vi "Write Coded Binary Data.vi"(7 "AC Data":refnum<class "Data.lvclass">, 8 "error in":errorcluster, 9 "cell":i32=-1, 10 "binRefIn":refnum<file>, 11 "PAS Cell Data in":refnum<class "PAS Cell Data.lvclass">) -> (0 "error out":errorcluster, 3 "PAS Cell Data out":refnum<class "PAS Cell Data.lvclass">)   [LabVIEW 2014, in "PAS Cell Data.lvclass"]
uses:
  PAS Cell Data.lvclass
  Data/Data.lvclass
  Main/Controls/Cell Data.ctl
  <vilib>/Analysis/Matrix/NI_Matrix.lvlib
  <vilib>/Analysis/Matrix/Numeric/Conversions/Matrix To Array - RM.vi
  Devices/Alicat/Data/MC/AlicatMCData.lvclass
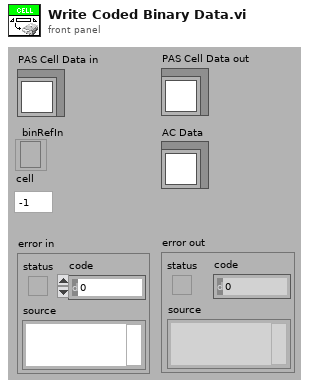
[diagram p1: front panel]
types:
  T1 = typedef "Cell Data.ctl" = u8
  T2 = enum16{"big-endian, network order", "native, host order", "little-endian"}
  T3 = typedef "NI_Matrix.lvlib/RealMatrix.ctl" = dbl[][]
  T4 = cluster{"P":sgl, "T":sgl, "Q":sgl, "Q0":sgl, "Qsp":sgl}
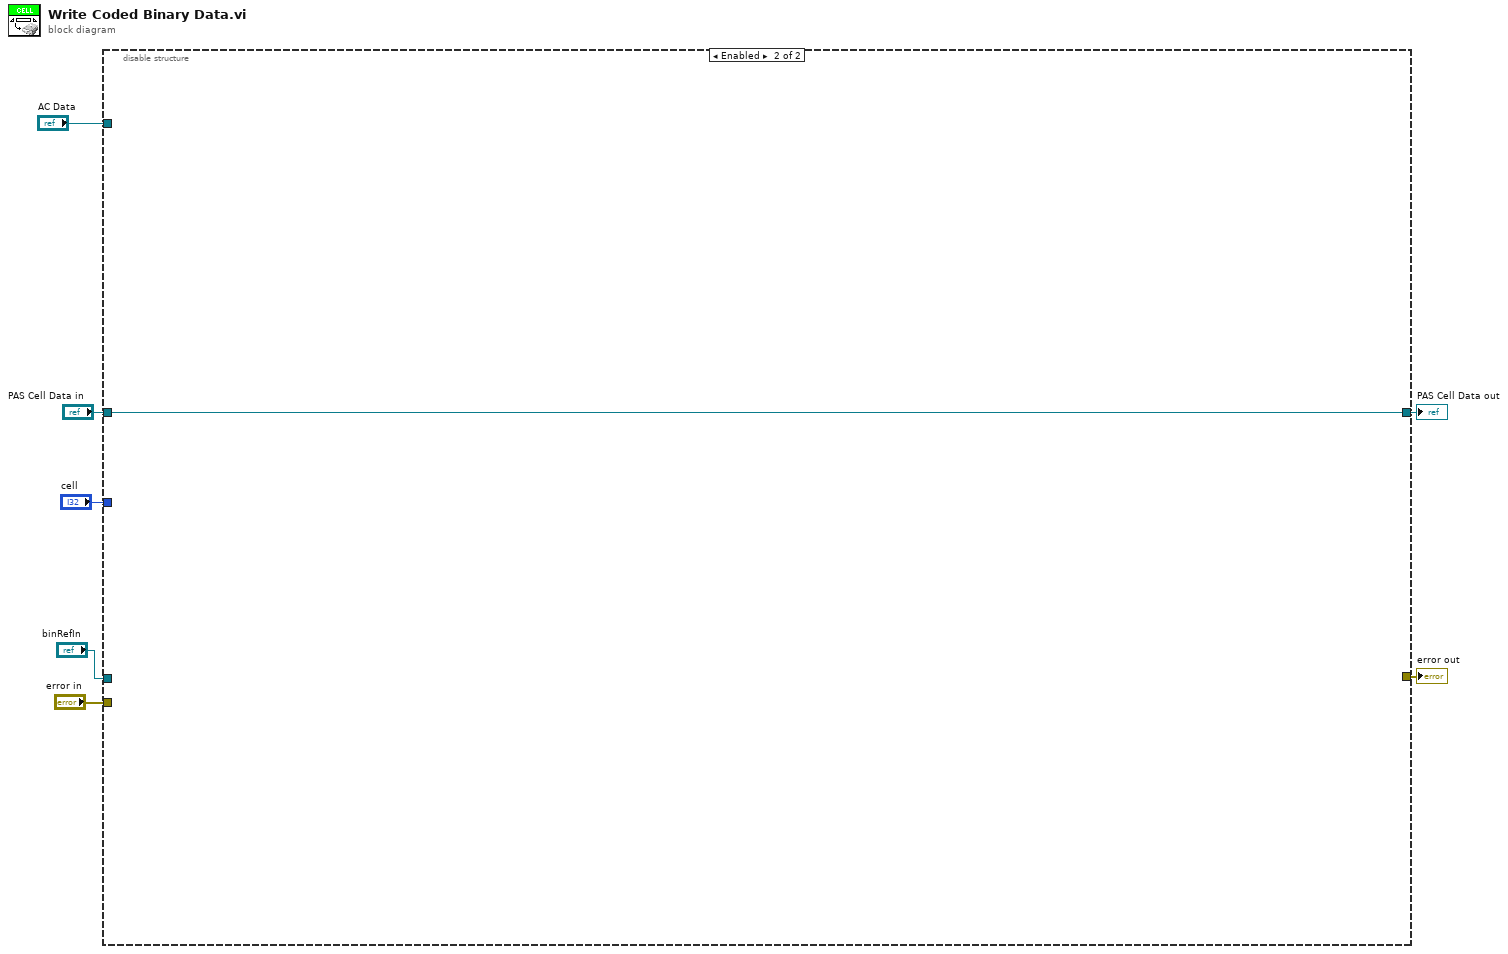
[diagram p0: block diagram]
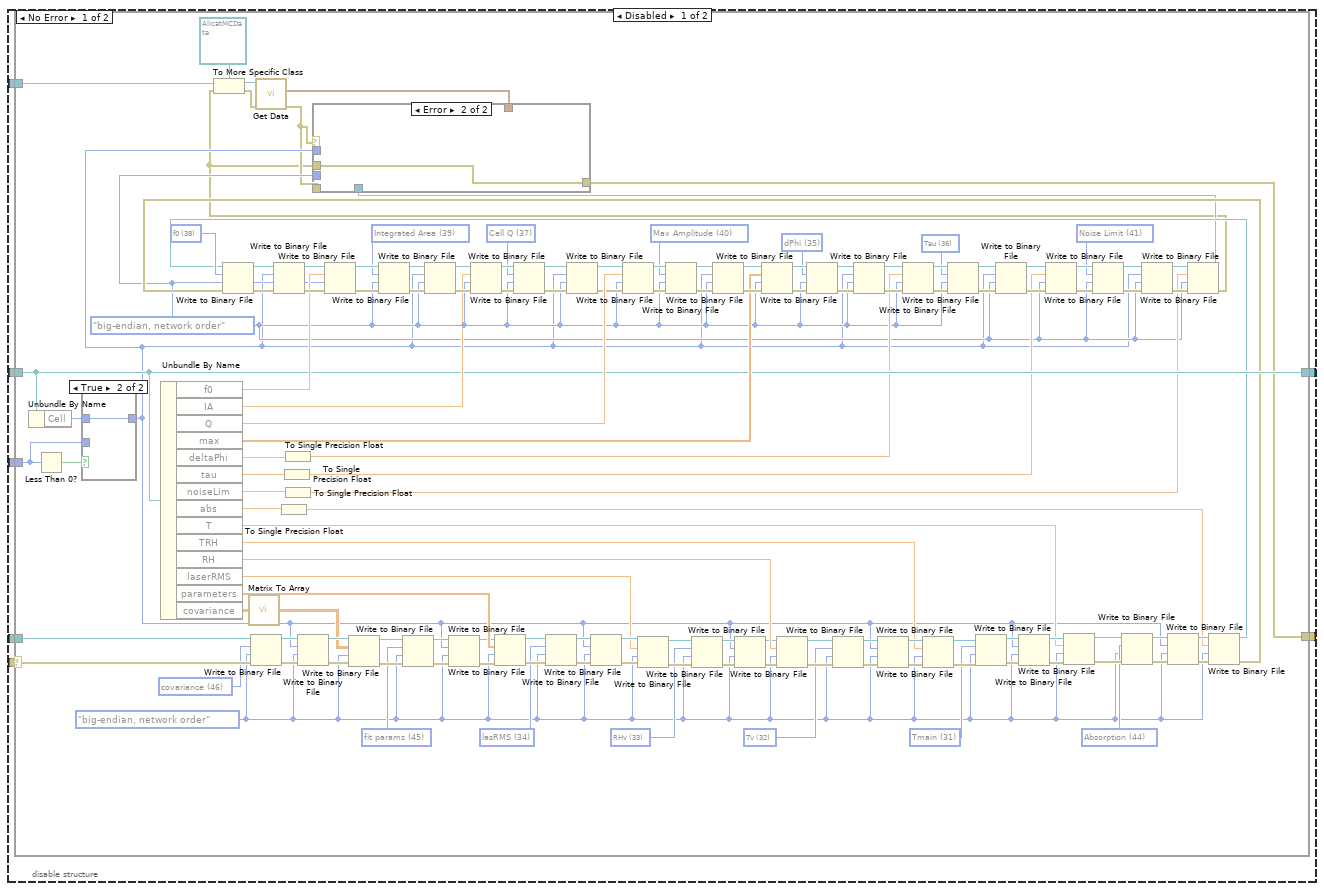
[diagram p2: hidden frame]
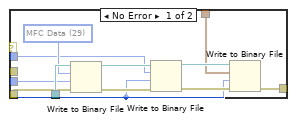
[diagram p3: hidden frame]
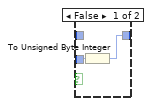
[diagram p4: hidden frame]
diagram:
  n1 = disable-structure shown="Enabled" {
    disable-tunnel: "error in" -> [w14 _]
    disable-tunnel: [w13 _] -> w6
    disable-tunnel: "PAS Cell Data in" -> [w12 w165]
    disable-tunnel: [w11 w165] -> w4
    disable-tunnel: "binRefIn" -> [w10 _]
    disable-tunnel: "cell" -> [w9 _]
    disable-tunnel: "AC Data" -> [w8 _]
    frame Disabled {
      n2 = case shown="No Error" w14 {
        selector: w14 -> [w147 w164]
        tunnel: [w19 w164] -> w13
        tunnel: [w39 w163] -> w11
        tunnel: w12 -> [w39 w163]
        tunnel: w10 -> [w55 _]
        tunnel: w9 -> [w27 _]
        tunnel: w8 -> [w24 _]
        frame No Error {
          w44 = T1 41 items=["TEC SP"=23, "TEC Enable"=24, "Qsp"=25, "Tac"=26, "Pac"=27, "Q0ac"=28, "Qac"=29, "Cell TEC T (T1)"=30, "Tmain"=31, "Tv"=32, "RHv"=33, "lasRMS"=34, "dPhi"=35, "Tau"=36, "Cell Q"=37, "f0"=38, "Integrated Area"=39, "Max Amplitude"=40, "Noise Limit"=41, "Lower Noise Bound"=42, "Upper Noise Bound"=43, "Absorption"=44, "fit params"=45, "covariance"=46] ("cellNumData")
          w45 = T1 36 items=["TEC SP"=23, "TEC Enable"=24, "Qsp"=25, "Tac"=26, "Pac"=27, "Q0ac"=28, "Qac"=29, "Cell TEC T (T1)"=30, "Tmain"=31, "Tv"=32, "RHv"=33, "lasRMS"=34, "dPhi"=35, "Tau"=36, "Cell Q"=37, "f0"=38, "Integrated Area"=39, "Max Amplitude"=40, "Noise Limit"=41, "Lower Noise Bound"=42, "Upper Noise Bound"=43, "Absorption"=44, "fit params"=45, "covariance"=46] ("cellNumData")
          w46 = T1 35 items=["TEC SP"=23, "TEC Enable"=24, "Qsp"=25, "Tac"=26, "Pac"=27, "Q0ac"=28, "Qac"=29, "Cell TEC T (T1)"=30, "Tmain"=31, "Tv"=32, "RHv"=33, "lasRMS"=34, "dPhi"=35, "Tau"=36, "Cell Q"=37, "f0"=38, "Integrated Area"=39, "Max Amplitude"=40, "Noise Limit"=41, "Lower Noise Bound"=42, "Upper Noise Bound"=43, "Absorption"=44, "fit params"=45, "covariance"=46] ("cellNumData")
          w48 = T1 40 items=["TEC SP"=23, "TEC Enable"=24, "Qsp"=25, "Tac"=26, "Pac"=27, "Q0ac"=28, "Qac"=29, "Cell TEC T (T1)"=30, "Tmain"=31, "Tv"=32, "RHv"=33, "lasRMS"=34, "dPhi"=35, "Tau"=36, "Cell Q"=37, "f0"=38, "Integrated Area"=39, "Max Amplitude"=40, "Noise Limit"=41, "Lower Noise Bound"=42, "Upper Noise Bound"=43, "Absorption"=44, "fit params"=45, "covariance"=46] ("cellNumData")
          w50 = T1 37 items=["TEC SP"=23, "TEC Enable"=24, "Qsp"=25, "Tac"=26, "Pac"=27, "Q0ac"=28, "Qac"=29, "Cell TEC T (T1)"=30, "Tmain"=31, "Tv"=32, "RHv"=33, "lasRMS"=34, "dPhi"=35, "Tau"=36, "Cell Q"=37, "f0"=38, "Integrated Area"=39, "Max Amplitude"=40, "Noise Limit"=41, "Lower Noise Bound"=42, "Upper Noise Bound"=43, "Absorption"=44, "fit params"=45, "covariance"=46] ("cellNumData")
          w52 = T1 39 items=["TEC SP"=23, "TEC Enable"=24, "Qsp"=25, "Tac"=26, "Pac"=27, "Q0ac"=28, "Qac"=29, "Cell TEC T (T1)"=30, "Tmain"=31, "Tv"=32, "RHv"=33, "lasRMS"=34, "dPhi"=35, "Tau"=36, "Cell Q"=37, "f0"=38, "Integrated Area"=39, "Max Amplitude"=40, "Noise Limit"=41, "Lower Noise Bound"=42, "Upper Noise Bound"=43, "Absorption"=44, "fit params"=45, "covariance"=46] ("cellNumData")
          w54 = T1 38 items=["TEC SP"=23, "TEC Enable"=24, "Qsp"=25, "Tac"=26, "Pac"=27, "Q0ac"=28, "Qac"=29, "Cell TEC T (T1)"=30, "Tmain"=31, "Tv"=32, "RHv"=33, "lasRMS"=34, "dPhi"=35, "Tau"=36, "Cell Q"=37, "f0"=38, "Integrated Area"=39, "Max Amplitude"=40, "Noise Limit"=41, "Lower Noise Bound"=42, "Upper Noise Bound"=43, "Absorption"=44, "fit params"=45, "covariance"=46] ("cellNumData")
          w18 = T2."big-endian, network order" ("byte order (0:big-endian, network order)")
          w93 = T1 44 items=["TEC SP"=23, "TEC Enable"=24, "Qsp"=25, "Tac"=26, "Pac"=27, "Q0ac"=28, "Qac"=29, "Cell TEC T (T1)"=30, "Tmain"=31, "Tv"=32, "RHv"=33, "lasRMS"=34, "dPhi"=35, "Tau"=36, "Cell Q"=37, "f0"=38, "Integrated Area"=39, "Max Amplitude"=40, "Noise Limit"=41, "Lower Noise Bound"=42, "Upper Noise Bound"=43, "Absorption"=44, "fit params"=45, "covariance"=46] ("cellNumData")
          w101 = T1 31 items=["TEC SP"=23, "TEC Enable"=24, "Qsp"=25, "Tac"=26, "Pac"=27, "Q0ac"=28, "Qac"=29, "Cell TEC T (T1)"=30, "Tmain"=31, "Tv"=32, "RHv"=33, "lasRMS"=34, "dPhi"=35, "Tau"=36, "Cell Q"=37, "f0"=38, "Integrated Area"=39, "Max Amplitude"=40, "Noise Limit"=41, "Lower Noise Bound"=42, "Upper Noise Bound"=43, "Absorption"=44, "fit params"=45, "covariance"=46] ("cellNumData")
          w109 = T1 32 items=["TEC SP"=23, "TEC Enable"=24, "Qsp"=25, "Tac"=26, "Pac"=27, "Q0ac"=28, "Qac"=29, "Cell TEC T (T1)"=30, "Tmain"=31, "Tv"=32, "RHv"=33, "lasRMS"=34, "dPhi"=35, "Tau"=36, "Cell Q"=37, "f0"=38, "Integrated Area"=39, "Max Amplitude"=40, "Noise Limit"=41, "Lower Noise Bound"=42, "Upper Noise Bound"=43, "Absorption"=44, "fit params"=45, "covariance"=46] ("cellNumData")
          w116 = T1 33 items=["TEC SP"=23, "TEC Enable"=24, "Qsp"=25, "Tac"=26, "Pac"=27, "Q0ac"=28, "Qac"=29, "Cell TEC T (T1)"=30, "Tmain"=31, "Tv"=32, "RHv"=33, "lasRMS"=34, "dPhi"=35, "Tau"=36, "Cell Q"=37, "f0"=38, "Integrated Area"=39, "Max Amplitude"=40, "Noise Limit"=41, "Lower Noise Bound"=42, "Upper Noise Bound"=43, "Absorption"=44, "fit params"=45, "covariance"=46] ("cellNumData")
          w125 = T1 34 items=["TEC SP"=23, "TEC Enable"=24, "Qsp"=25, "Tac"=26, "Pac"=27, "Q0ac"=28, "Qac"=29, "Cell TEC T (T1)"=30, "Tmain"=31, "Tv"=32, "RHv"=33, "lasRMS"=34, "dPhi"=35, "Tau"=36, "Cell Q"=37, "f0"=38, "Integrated Area"=39, "Max Amplitude"=40, "Noise Limit"=41, "Lower Noise Bound"=42, "Upper Noise Bound"=43, "Absorption"=44, "fit params"=45, "covariance"=46] ("cellNumData")
          w92 = T2."big-endian, network order" ("byte order (0:big-endian, network order)")
          w135 = T1 45 items=["TEC SP"=23, "TEC Enable"=24, "Qsp"=25, "Tac"=26, "Pac"=27, "Q0ac"=28, "Qac"=29, "Cell TEC T (T1)"=30, "Tmain"=31, "Tv"=32, "RHv"=33, "lasRMS"=34, "dPhi"=35, "Tau"=36, "Cell Q"=37, "f0"=38, "Integrated Area"=39, "Max Amplitude"=40, "Noise Limit"=41, "Lower Noise Bound"=42, "Upper Noise Bound"=43, "Absorption"=44, "fit params"=45, "covariance"=46] ("cellNumData")
          w145 = T1 46 items=["TEC SP"=23, "TEC Enable"=24, "Qsp"=25, "Tac"=26, "Pac"=27, "Q0ac"=28, "Qac"=29, "Cell TEC T (T1)"=30, "Tmain"=31, "Tv"=32, "RHv"=33, "lasRMS"=34, "dPhi"=35, "Tau"=36, "Cell Q"=37, "f0"=38, "Integrated Area"=39, "Max Amplitude"=40, "Noise Limit"=41, "Lower Noise Bound"=42, "Upper Noise Bound"=43, "Absorption"=44, "fit params"=45, "covariance"=46] ("cellNumData")
          n3 = Unbundle By Name(w39) -> ("Cell"=w26:u8)
          n4 = Less Than 0?(x=w27) -> (x < 0?=w28:bool)
          n5 = case shown="True" w28 {
            tunnel: w27 -> [w161 _]
            tunnel: [w160 w162] -> w17
            tunnel: w26 -> [_ w162]
            frame False {
              n6 = To Unsigned Byte Integer(number=w161) -> (unsigned 8bit integer=w160:u8)
            }
            frame True {
            }
          }
          n7 = Unbundle By Name(w39) -> ("f0"=w53:sgl, "IA"=w51:sgl, "Q"=w49:sgl, "max"=w47:dbl[], "deltaPhi"=w30:dbl, "tau"=w32:dbl, "noiseLim"=w34:dbl, "abs"=w36:dbl, "T"=w100:sgl, "TRH"=w108:sgl, "RH"=w123:sgl, "laserRMS"=w124:sgl, "parameters"=w134:dbl[], "covariance"=w146:T3)
          n8 = call-poly <vilib>:"Matrix To Array.vi"("Real Matrix"=w146) -> ("Real 2D Array"=w136:dbl[][])
          n9 = Write to Binary File(file (use dialog)=w55, data=w145, error in=w147, 9:w92) -> (refnum out=w143:refnum<file>, error out=w144:errorcluster)  [unwired: 2 in, 1 out]
          n10 = To Single Precision Float(number=w36) -> (single precision float=w35:sgl)
          n11 = To Single Precision Float(number=w32) -> (single precision float=w31:sgl)
          n12 = To Single Precision Float(number=w30) -> (single precision float=w29:sgl)
          n13 = To Single Precision Float(number=w34) -> (single precision float=w33:sgl)
          n14 = Write to Binary File(file (use dialog)=w143, data=w17, error in=w144, 9:w92) -> (refnum out=w142:refnum<file>, error out=w141:errorcluster)  [unwired: 2 in, 1 out]
          n15 = Write to Binary File(file (use dialog)=w142, data=w136, error in=w141, 9:w92) -> (refnum out=w140:refnum<file>, error out=w139:errorcluster)  [unwired: 2 in, 1 out]
          n16 = Write to Binary File(file (use dialog)=w140, data=w135, error in=w139, 9:w92) -> (refnum out=w138:refnum<file>, error out=w137:errorcluster)  [unwired: 2 in, 1 out]
          n17 = Write to Binary File(file (use dialog)=w138, data=w17, error in=w137, 9:w92) -> (refnum out=w133:refnum<file>, error out=w132:errorcluster)  [unwired: 2 in, 1 out]
          n18 = Write to Binary File(file (use dialog)=w133, data=w134, error in=w132, 9:w92) -> (refnum out=w131:refnum<file>, error out=w130:errorcluster)  [unwired: 2 in, 1 out]
          n19 = Write to Binary File(file (use dialog)=w131, data=w125, error in=w130, 9:w92) -> (refnum out=w129:refnum<file>, error out=w128:errorcluster)  [unwired: 2 in, 1 out]
          n20 = Write to Binary File(file (use dialog)=w129, data=w17, error in=w128, 9:w92) -> (refnum out=w127:refnum<file>, error out=w126:errorcluster)  [unwired: 2 in, 1 out]
          n21 = Write to Binary File(file (use dialog)=w127, data=w124, error in=w126, 9:w92) -> (refnum out=w122:refnum<file>, error out=w121:errorcluster)  [unwired: 2 in, 1 out]
          n22 = Write to Binary File(file (use dialog)=w122, data=w116, error in=w121, 9:w92) -> (refnum out=w120:refnum<file>, error out=w119:errorcluster)  [unwired: 2 in, 1 out]
          n23 = Write to Binary File(file (use dialog)=w120, data=w17, error in=w119, 9:w92) -> (refnum out=w118:refnum<file>, error out=w117:errorcluster)  [unwired: 2 in, 1 out]
          n24 = Write to Binary File(file (use dialog)=w118, data=w123, error in=w117, 9:w92) -> (refnum out=w114:refnum<file>, error out=w115:errorcluster)  [unwired: 2 in, 1 out]
          n25 = Write to Binary File(file (use dialog)=w114, data=w109, error in=w115, 9:w92) -> (refnum out=w112:refnum<file>, error out=w113:errorcluster)  [unwired: 2 in, 1 out]
          n26 = Write to Binary File(file (use dialog)=w112, data=w17, error in=w113, 9:w92) -> (refnum out=w110:refnum<file>, error out=w111:errorcluster)  [unwired: 2 in, 1 out]
          n27 = Write to Binary File(file (use dialog)=w110, data=w108, error in=w111, 9:w92) -> (refnum out=w106:refnum<file>, error out=w107:errorcluster)  [unwired: 2 in, 1 out]
          n28 = Write to Binary File(file (use dialog)=w106, data=w101, error in=w107, 9:w92) -> (refnum out=w105:refnum<file>, error out=w104:errorcluster)  [unwired: 2 in, 1 out]
          n29 = Write to Binary File(file (use dialog)=w105, data=w17, error in=w104, 9:w92) -> (refnum out=w103:refnum<file>, error out=w102:errorcluster)  [unwired: 2 in, 1 out]
          n30 = Write to Binary File(file (use dialog)=w103, data=w100, error in=w102, 9:w92) -> (refnum out=w99:refnum<file>, error out=w98:errorcluster)  [unwired: 2 in, 1 out]
          n31 = Write to Binary File(file (use dialog)=w99, data=w93, error in=w98, 9:w92) -> (refnum out=w97:refnum<file>, error out=w96:errorcluster)  [unwired: 2 in, 1 out]
          n32 = Write to Binary File(file (use dialog)=w97, data=w17, error in=w96, 9:w92) -> (refnum out=w95:refnum<file>, error out=w94:errorcluster)  [unwired: 2 in, 1 out]
          n33 = Write to Binary File(file (use dialog)=w95, data=w35, error in=w94, 9:w92) -> (refnum out=w38:refnum<file>, error out=w37:errorcluster)  [unwired: 2 in, 1 out]
          n34 = Write to Binary File(file (use dialog)=w38, data=w54, error in=w37, 9:w18) -> (refnum out=w57:refnum<file>, error out=w56:errorcluster)  [unwired: 2 in, 1 out]
          n35 = Write to Binary File(file (use dialog)=w57, data=w17, error in=w56, 9:w18) -> (refnum out=w58:refnum<file>, error out=w59:errorcluster)  [unwired: 2 in, 1 out]
          n36 = Write to Binary File(file (use dialog)=w58, data=w53, error in=w59, 9:w18) -> (refnum out=w60:refnum<file>, error out=w61:errorcluster)  [unwired: 2 in, 1 out]
          n37 = Write to Binary File(file (use dialog)=w60, data=w52, error in=w61, 9:w18) -> (refnum out=w62:refnum<file>, error out=w63:errorcluster)  [unwired: 2 in, 1 out]
          n38 = Write to Binary File(file (use dialog)=w62, data=w17, error in=w63, 9:w18) -> (refnum out=w64:refnum<file>, error out=w65:errorcluster)  [unwired: 2 in, 1 out]
          n39 = Write to Binary File(file (use dialog)=w64, data=w51, error in=w65, 9:w18) -> (refnum out=w66:refnum<file>, error out=w67:errorcluster)  [unwired: 2 in, 1 out]
          n40 = Write to Binary File(file (use dialog)=w66, data=w50, error in=w67, 9:w18) -> (refnum out=w42:refnum<file>, error out=w43:errorcluster)  [unwired: 2 in, 1 out]
          n41 = Write to Binary File(file (use dialog)=w42, data=w17, error in=w43, 9:w18) -> (refnum out=w41:refnum<file>, error out=w40:errorcluster)  [unwired: 2 in, 1 out]
          n42 = Write to Binary File(file (use dialog)=w41, data=w49, error in=w40, 9:w18) -> (refnum out=w68:refnum<file>, error out=w69:errorcluster)  [unwired: 2 in, 1 out]
          n43 = Write to Binary File(file (use dialog)=w68, data=w48, error in=w69, 9:w18) -> (refnum out=w70:refnum<file>, error out=w71:errorcluster)  [unwired: 2 in, 1 out]
          n44 = Write to Binary File(file (use dialog)=w70, data=w17, error in=w71, 9:w18) -> (refnum out=w72:refnum<file>, error out=w73:errorcluster)  [unwired: 2 in, 1 out]
          n45 = Write to Binary File(file (use dialog)=w72, data=w47, error in=w73, 9:w18) -> (refnum out=w74:refnum<file>, error out=w75:errorcluster)  [unwired: 2 in, 1 out]
          n46 = Write to Binary File(file (use dialog)=w74, data=w46, error in=w75, 9:w18) -> (refnum out=w77:refnum<file>, error out=w76:errorcluster)  [unwired: 2 in, 1 out]
          n47 = Write to Binary File(file (use dialog)=w77, data=w17, error in=w76, 9:w18) -> (refnum out=w79:refnum<file>, error out=w78:errorcluster)  [unwired: 2 in, 1 out]
          n48 = Write to Binary File(file (use dialog)=w79, data=w29, error in=w78, 9:w18) -> (refnum out=w81:refnum<file>, error out=w80:errorcluster)  [unwired: 2 in, 1 out]
          n49 = Write to Binary File(file (use dialog)=w81, data=w45, error in=w80, 9:w18) -> (refnum out=w83:refnum<file>, error out=w82:errorcluster)  [unwired: 2 in, 1 out]
          n50 = Write to Binary File(file (use dialog)=w83, data=w17, error in=w82, 9:w18) -> (refnum out=w84:refnum<file>, error out=w85:errorcluster)  [unwired: 2 in, 1 out]
          n51 = Write to Binary File(file (use dialog)=w84, data=w31, error in=w85, 9:w18) -> (refnum out=w86:refnum<file>, error out=w87:errorcluster)  [unwired: 2 in, 1 out]
          n52 = Write to Binary File(file (use dialog)=w86, data=w44, error in=w87, 9:w18) -> (refnum out=w88:refnum<file>, error out=w89:errorcluster)  [unwired: 2 in, 1 out]
          n53 = Write to Binary File(file (use dialog)=w88, data=w17, error in=w89, 9:w18) -> (refnum out=w90:refnum<file>, error out=w91:errorcluster)  [unwired: 2 in, 1 out]
          n54 = Write to Binary File(file (use dialog)=w90, data=w33, error in=w91, 9:w18) -> (refnum out=w21:refnum<file>, error out=w15:errorcluster)  [unwired: 2 in, 1 out]
          n55 = To More Specific Class(target class=refnum<class "AlicatMCData.lvclass"> refnum ("Alicat.lvlib:AlicatMCData.lvclass"), reference=w24, error in=w15) -> (specific class reference=w25:refnum<class "AlicatMCData.lvclass">, error out=w22:errorcluster)
          n56 = call "Get Data.vi"("error in"=w22, "AlicatMData in"=w25) -> ("error out"=w16:errorcluster, "SystemData"=w20:T4)  [unwired: 7 in, 1 out]
          n57 = case shown="Error" w16 {
            tunnel: w21 -> [w158 _]
            tunnel: w16 -> [w155 _]
            tunnel: w20 -> [w152 _]
            tunnel: [w151 w159] -> w19
            tunnel: w18 -> [w150 _]
            tunnel: w17 -> [w148 _]
            tunnel: w15 -> [_ w159]
            frame No Error {
              w149 = T1 29 items=["TEC SP"=23, "TEC Enable"=24, "MFC Data"=29, "Cell TEC T (T1)"=30, "Tmain"=31, "Tv"=32, "RHv"=33, "lasRMS"=34, "dPhi"=35, "Tau"=36, "Cell Q"=37, "f0"=38, "Integrated Area"=39, "Max Amplitude"=40, "Noise Limit"=41, "Lower Noise Bound"=42, "Upper Noise Bound"=43, "Absorption"=44, "fit params"=45, "covariance"=46] ("cellNumData")
              n58 = Write to Binary File(file (use dialog)=w158, data=w149, error in=w155, 9:w150) -> (refnum out=w157:refnum<file>, error out=w156:errorcluster)  [unwired: 2 in, 1 out]
              n59 = Write to Binary File(file (use dialog)=w157, data=w148, error in=w156, 9:w150) -> (refnum out=w154:refnum<file>, error out=w153:errorcluster)  [unwired: 2 in, 1 out]
              n60 = Write to Binary File(file (use dialog)=w154, data=w152, error in=w153, 9:w150) -> (error out=w151:errorcluster)  [unwired: 2 in, 2 out]
            }
            frame Error {
            }
          }
        }
        frame Error {
        }
      }
    }
    frame Enabled {
    }
  }
  "error out" <- w6
  "PAS Cell Data out" <- w4
